vi "Write Variant (dyn prop).vi"(8 "error in (no error)":errorcluster, 10 "Variant":variant, 11 "Test Object in":refnum<class "Test Object.lvclass">) -> (0 "error out":errorcluster, 3 "Test Object out":refnum<class "Test Object.lvclass">)   [LabVIEW 2015, in "Test Object.lvclass"]
uses:
  Test Object.lvclass
  Test Object.lvclass/Test Object.ctl
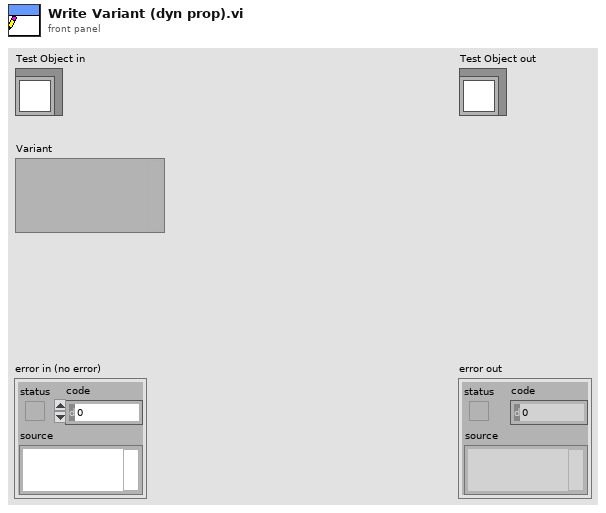
[diagram p1: front panel]
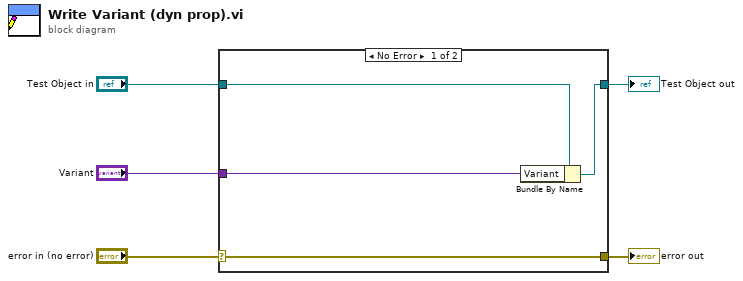
[diagram p0: block diagram]
diagram:
  n1 = case shown="No Error" "error in (no error)" {
    selector: "error in (no error)" -> [w9 w10]
    tunnel: [w9 w10] -> w4
    tunnel: [w7 w11] -> w2
    tunnel: "Test Object in" -> [w8 w11]
    tunnel: "Variant" -> [w6 _]
    frame No Error {
      n2 = Bundle By Name(cluster=w8, "Variant"=w6) -> (w7:refnum<class "Test Object.lvclass">)
    }
    frame Error {
    }
  }
  "error out" <- w4
  "Test Object out" <- w2
